vi "fgv_고장진단_config.vi"(7 "cmd":T2, 11 "고장진단 기준 값":T1) -> (3 "고장진단 기준 값 2":T1)   [LabVIEW 2019]
uses:
  _ctrl/rw.ctl
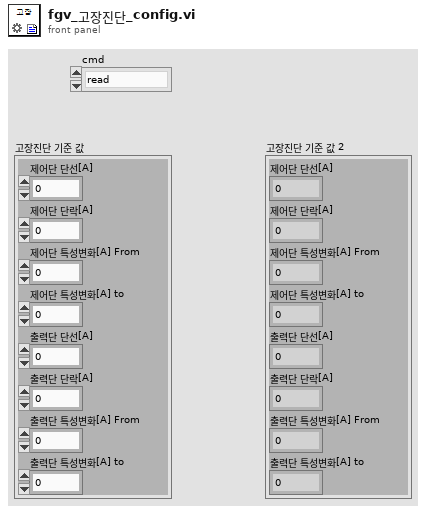
[diagram p1: front panel]
types:
  T1 = cluster{"제어단 단선[A]":dbl, "제어단 단락[A]":dbl, "제어단 특성변화[A] From":dbl, "제어단 특성변화[A] to":dbl, "출력단 단선[A]":dbl, "출력단 단락[A]":dbl, "출력단 특성변화[A] From":dbl, "출력단 특성변화[A] to":dbl}
  T2 = typedef "rw.ctl" = enum16{"read", "write"}
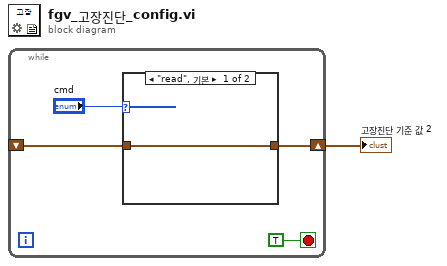
[diagram p0: block diagram]
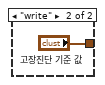
[diagram p2: hidden frame]
diagram:
  n1 = while {
    shift-right: [w4] -> w1
    shift-left: _ -> [w3]
    stop <- TRUE stop-if-true
    n2 = case shown="\"read\", 기본" "cmd" {
      tunnel: [w6 "고장진단 기준 값"] -> w4
      tunnel: w3 -> [w6 _]
      frame "read", Default {
      }
      frame "write" {
      }
    }
  }
  "고장진단 기준 값 2" <- w1
